vi "Set Image.vi"(5 "vend":i32, 6 "vstart":i32, 7 "hend":i32, 8 "error in (no error)":errorcluster, 9 "hstart":i32, 10 "vbin":i32, 11 "hbin":i32) -> (0 "error out":errorcluster, 3 "function return":u32)   [LabVIEW 2014, in "atmcd32d.lvlib"]
doc: "unsigned int WINAPI SetImage(int hbin, int vbin, int hstart, int hend, int vstart, int vend);"
uses:
  atmcd32d.lvlib
  atmcd32d.dll
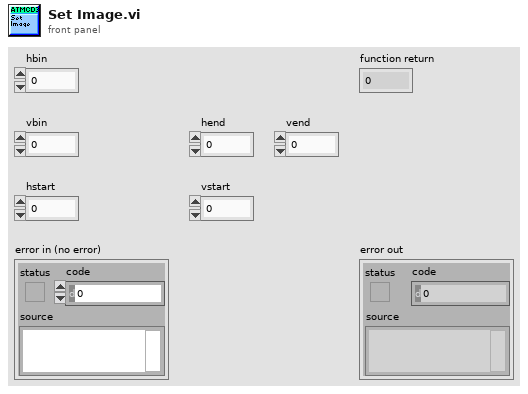
[diagram p1: front panel]
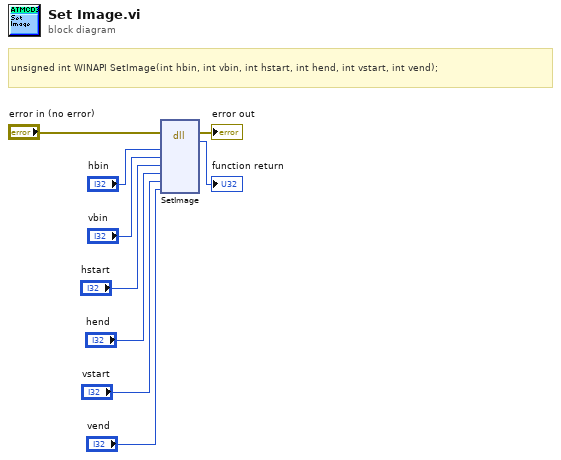
[diagram p0: block diagram]
diagram:
  # "unsigned int WINAPI SetImage(int hbin, int vbin, int hstart, int hend, int vstart, int vend);"
  n1 = dll-call lib="C:/Users/Bakir/Documents/Lambda2-Testing/lib/Andorlib/atmcd32d.*" fn="SetImage"(error in="error in (no error)", "hbin"="hbin", "vbin"="vbin", "hstart"="hstart", "hend"="hend", "vstart"="vstart", "vend"="vend") -> (error out=→"error out":errorcluster, →"function return":u32)  [unwired: 8 in, 1 out]
